vi "Configure A to B Sequence Trigger.vi"(0 "VISA resource name":refnum<visa-resource-name>, 1 "Enable B Trigger (T: Enable)":bool=TRUE, 2 "Trigger Reset Type (0:None)":u16(ring) items=["None", "Timeout", "State (Low)", "State (High)", "Transition (Rising)", "Transition (Falling)"], 5 "Trigger Mode (0:Trig After Time)":u16(ring) items=["Trig After Time", "Trig On nth Event"], 7 "Trigger Delay Time (6.0ns)":dbl=6e-09, 9 "Trigger Event (1)":i32=1, 11 "error in (no error)":errorcluster, 12 "Timeout (1.0Ms)":dbl=1000000.0, 13 "Source (0:Channel1)":u16(ring) items=["Channel1"=0, "Channel2"=1, "Channel3"=2, "Channel4"=3, "Aux"=12], 14 "Threshold (0.0v)":dbl) -> (4 "VISA resource name out":refnum<visa-resource-name>, 15 "error out":errorcluster)   [LabVIEW 2015, in "Tektronix 7000 Series.lvlib"]
doc: "Configures A to B Sequence. B trigger occurs after the main trigger event. It is available only when you enable B Trigger Type.\n\n<B>Note:</B> Not all models support all parameters contained in this VI. These settings are ignored by the driver if not supported.\n\nThis VI has been obsoleted from the driver and is included for compatibility with existing applications. New applications should use the Configure Trigger (A to B Sequence Mode) VI"
uses:
  <instrlib>/Tektronix 7000 Series/Tektronix 7000 Series.lvlib
panel:
  # "Note:\nThis VI has been obsoleted from the driver and is included for compatibility with existing applications.  New applications should use the Configure Trigger (A to B Sequence Mode) VI"
  # "Trigger Reset"
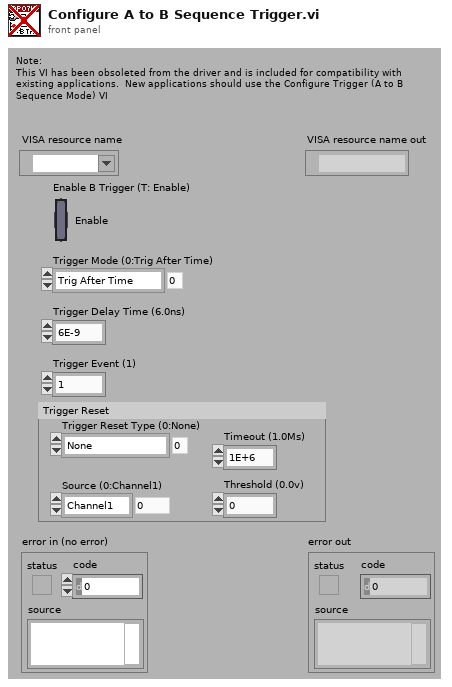
[diagram p1: front panel]
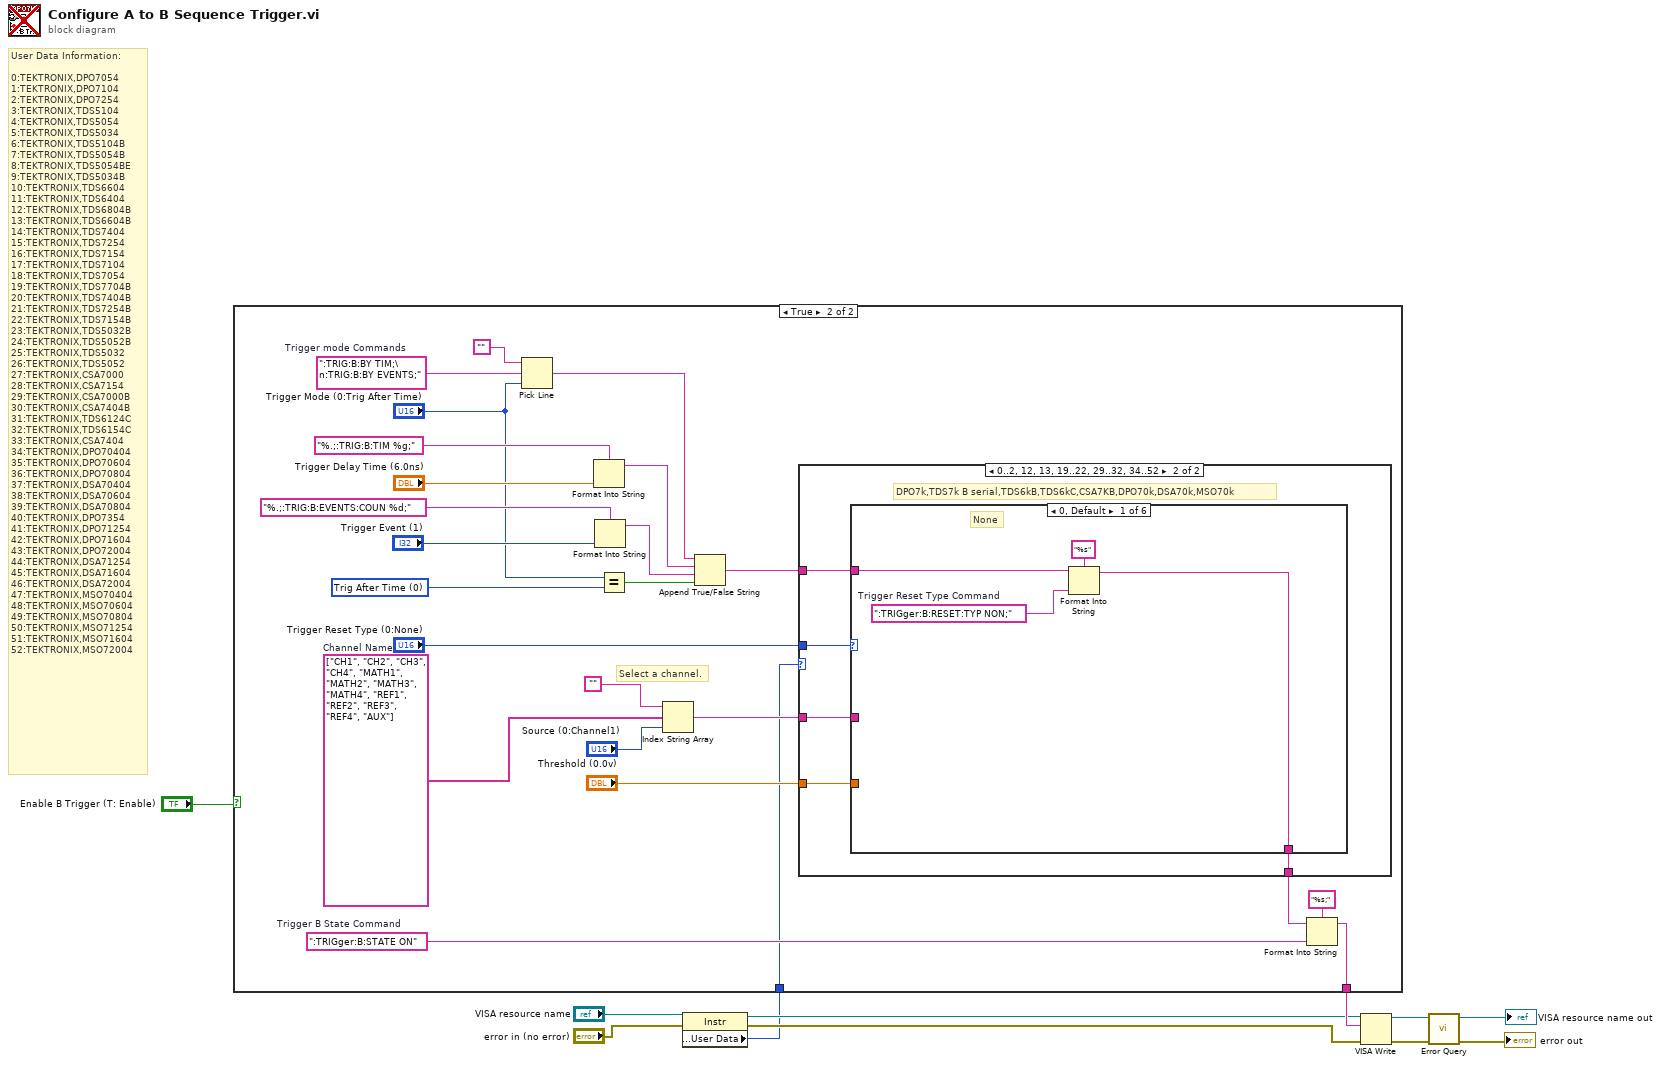
[diagram p0: block diagram]
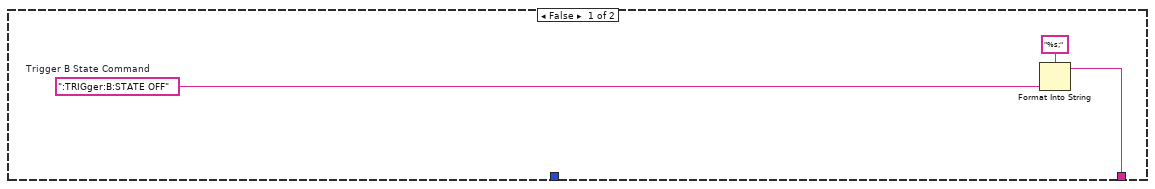
[diagram p2: hidden frame]
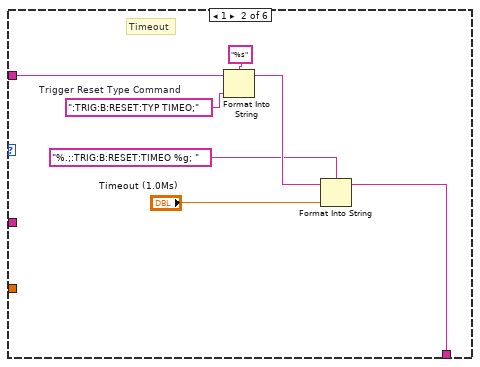
[diagram p4: hidden frame]
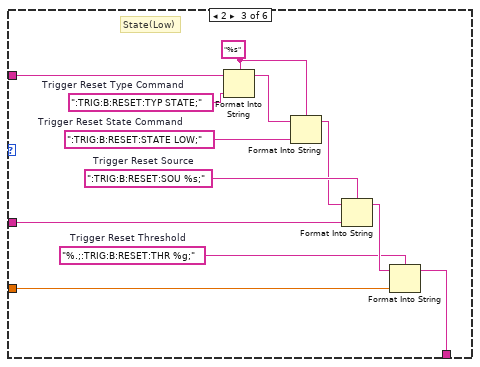
[diagram p5: hidden frame]
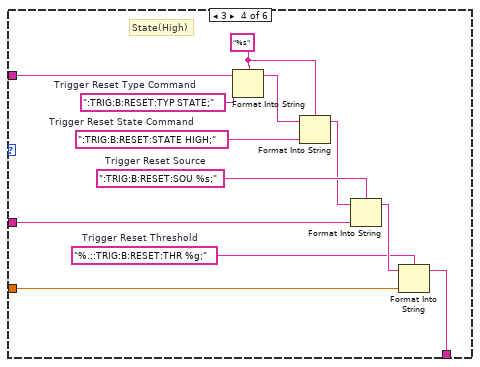
[diagram p6: hidden frame]
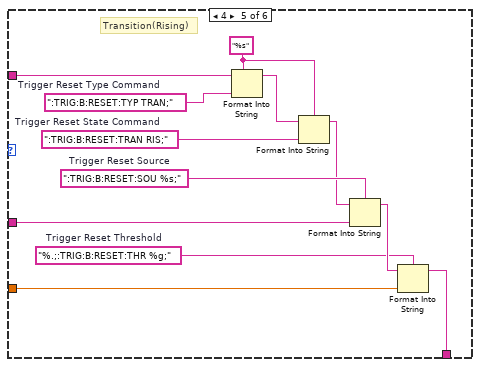
[diagram p7: hidden frame]
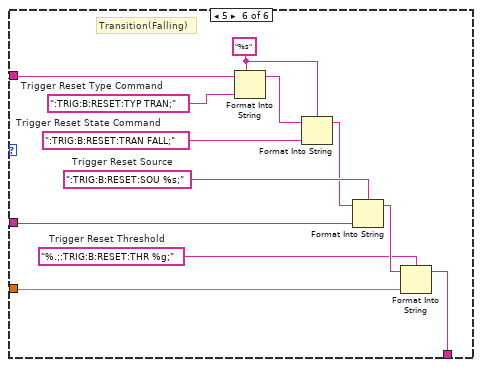
[diagram p8: hidden frame]
diagram:
  # "User Data Information:\n\n0:TEKTRONIX,DPO7054\n1:TEKTRONIX,DPO7104\n2:TEKTRONIX,DPO7254\n3:TEKTRONIX,TDS5104\n4:TEKTRONIX,TDS5054\n5:TEKTRONIX,TDS5034\n6:TEKTRONIX,TDS5104B\n7:TEKTRONIX,TDS5054B\n8:TEKTRONIX,TDS5054BE\n9:TEKTRONIX,TDS5034B\n10:TEKTRONIX,TDS6604\n11:TEKTRONIX,TDS6404\n12:TEKTRONIX,TDS6804B\n13:TEKTRONIX,TDS6604B\n14:TEKTRONIX,TDS7404\n15:TEKTRONIX,TDS7254\n16:TEKTRONIX,TDS7154\n17:TEKTRONIX,TDS7104\n18:TEKTRONIX,TDS7054\n19:TEKTRONIX,TDS7704B\n20:TEKTRONIX,TDS7404B\n21:TEKTRONIX,TDS7254B\n22:TEKTRONIX,TDS7154B\n23:TEKTRONIX,TDS5032B\n24:TEKTRONIX,TDS5052B\n25:TEKTRONIX,TDS5032\n26:TEKTRONIX,TDS5052\n27:TEKTRONIX,CSA7000\n28:TEKTRONIX,CSA7154\n29:TEKTRONIX,CSA7000B\n30:TEKTRONIX,CSA7404B\n31:TEKTRONIX,TDS6124C\n32:TEKTRONIX,TDS6154C\n33:TEKTRONIX,CSA7404\n34:TEKTRONIX,DPO70404\n35:TEKTRONIX,DPO70604\n36:TEKTRONIX,DPO70804\n37:TEKTRONIX,DSA70404\n38:TEKTRONIX,DSA70604\n39:TEKTRONIX,DSA70804\n40:TEKTRONIX,DPO7354\n41:TEKTRONIX,DPO71254\n42:TEKTRONIX,DPO71604\n43:TEKTRONIX,DPO72004\n44:TEKTRONIX,DSA71254\n45:TEKTRONIX,DSA71604\n46:TEKTRONIX,DSA72004\n47:TEKTRONIX,MSO70404\n48:TEKTRONIX,MSO70604\n49:TEKTRONIX,MSO70804\n50:TEKTRONIX,MSO71254\n51:TEKTRONIX,MSO71604\n52:TEKTRONIX,MSO72004"
  n1 = property class="Instr"(reference="VISA resource name", error in="error in (no error)") -> (reference out=w3:refnum<visa-resource-name>, error out=w2:errorcluster, "General Settings:User Data"=w1:u32)
  n2 = case shown="True" "Enable B Trigger (T: Enable)" {
    tunnel: [w12 w16] -> w7
    tunnel: w1 -> [_ w15]
    frame False {
      w14 = ":TRIGger:B:STATE OFF"  # Trigger B State Command
      n3 = Format Into String(format string="%s;", w14) -> (resulting string=w12:string)  [unwired: 2 in, 1 out]
    }
    frame True {
      w18 = ":TRIGger:B:STATE ON"  # Trigger B State Command
      w24 = string[] ["CH1", "CH2", "CH3", "CH4", "MATH1", "MATH2", "MATH3", "MATH4", "REF1", "REF2", "REF3", "REF4", "AUX"]  # Channel Name
      w32 = u16 0 items=["Trig After Time", "Trig On nth Event"] ("Trigger mode (0:Trig After Time)")
      w38 = ":TRIG:B:BY TIM;\n:TRIG:B:BY EVENTS;"  # Trigger mode Commands
      # "Select a channel."
      n4 = Pick Line(string ("")="" ("Empty String Constant"), multi-line string=w38, line index="Trigger Mode (0:Trig After Time)") -> (output string=w27:string)
      n5 = Format Into String(format string="%.;:TRIG:B:TIM %g;", "Trigger Delay Time (6.0ns)") -> (resulting string=w29:string)  [unwired: 2 in, 1 out]
      n6 = Format Into String(format string="%.;:TRIG:B:EVENTS:COUN %d;", "Trigger Event (1)") -> (resulting string=w28:string)  [unwired: 2 in, 1 out]
      n7 = Equal?(x="Trigger Mode (0:Trig After Time)", y=w32) -> (x = y?=w30:bool)
      n8 = Index String Array(1:"Source (0:Channel1)", 2:w24, 3:"" ("Empty String Constant")) -> (0:w21:string)
      n9 = Append True/False String(1:w30, 2:w28, 3:w29, 4:w27) -> (0:w25:string)
      n10 = case shown="0..2, 12, 13, 19..22, 29..32, 34..52" w15 {
        tunnel: "Trigger Reset Type (0:None)" -> [_ w44]
        tunnel: w25 -> [w39 w43]
        tunnel: w21 -> [_ w42]
        tunnel: "Threshold (0.0v)" -> [_ w41]
        tunnel: [w39 w40] -> w17
        frame Default {
        }
        frame 0..2, 12, 13, 19..22, 29..32, 34..52 {
          # "DPO7k,TDS7k B serial,TDS6kB,TDS6kC,CSA7KB,DPO70k,DSA70k,MSO70k"
          n11 = case shown="0, Default" w44 {
            tunnel: w43 -> [w47 w52 w66 w73 w83 w94]
            tunnel: w42 -> [_ _ w61 w72 w81 w93]
            tunnel: w41 -> [_ _ w58 w71 w82 w95]
            tunnel: [w45 w49 w56 w69 w80 w92] -> w40
            frame 0, Default {
              w46 = ":TRIGger:B:RESET:TYP NON;"  # Trigger Reset Type Command
              # "None"
              n12 = Format Into String(format string="%s", initial string=w47, w46) -> (resulting string=w45:string)  [unwired: 1 in, 1 out]
            }
            frame 1 {
              w53 = ":TRIG:B:RESET:TYP TIMEO;"  # Trigger Reset Type Command
              # "Timeout"
              n13 = Format Into String(format string="%s", initial string=w52, w53) -> (resulting string=w51:string)  [unwired: 1 in, 1 out]
              n14 = Format Into String(format string="%.;:TRIG:B:RESET:TIMEO %g; ", initial string=w51, "Timeout (1.0Ms)") -> (resulting string=w49:string)  [unwired: 1 in, 1 out]
            }
            frame 2 {
              w57 = "%.;:TRIG:B:RESET:THR %g;"  # Trigger Reset Threshold
              w64 = ":TRIG:B:RESET:STATE LOW;"  # Trigger Reset State Command
              w62 = ":TRIG:B:RESET:SOU %s;"  # Trigger Reset Source
              w65 = "%s" ("format string")
              w67 = ":TRIG:B:RESET:TYP STATE;"  # Trigger Reset Type Command
              # "State(Low)"
              n15 = Format Into String(format string=w65, initial string=w66, w67) -> (resulting string=w63:string)  [unwired: 1 in, 1 out]
              n16 = Format Into String(format string=w65, initial string=w63, w64) -> (resulting string=w60:string)  [unwired: 1 in, 1 out]
              n17 = Format Into String(format string=w62, initial string=w60, w61) -> (resulting string=w59:string)  [unwired: 1 in, 1 out]
              n18 = Format Into String(format string=w57, initial string=w59, w58) -> (resulting string=w56:string)  [unwired: 1 in, 1 out]
            }
            frame 3 {
              w74 = "%.;:TRIG:B:RESET:THR %g;"  # Trigger Reset Threshold
              w79 = ":TRIG:B:RESET:STATE HIGH;"  # Trigger Reset State Command
              w77 = ":TRIG:B:RESET:SOU %s;"  # Trigger Reset Source
              w70 = "%s" ("format string")
              w68 = ":TRIG:B:RESET:TYP STATE;"  # Trigger Reset Type Command
              # "State(High)"
              n19 = Format Into String(format string=w70, initial string=w73, w68) -> (resulting string=w78:string)  [unwired: 1 in, 1 out]
              n20 = Format Into String(format string=w70, initial string=w78, w79) -> (resulting string=w76:string)  [unwired: 1 in, 1 out]
              n21 = Format Into String(format string=w77, initial string=w76, w72) -> (resulting string=w75:string)  [unwired: 1 in, 1 out]
              n22 = Format Into String(format string=w74, initial string=w75, w71) -> (resulting string=w69:string)  [unwired: 1 in, 1 out]
            }
            frame 4 {
              w84 = "%.;:TRIG:B:RESET:THR %g;"  # Trigger Reset Threshold
              w89 = ":TRIG:B:RESET:TRAN RIS;"  # Trigger Reset State Command
              w87 = ":TRIG:B:RESET:SOU %s;"  # Trigger Reset Source
              w91 = "%s" ("format string")
              w90 = ":TRIG:B:RESET:TYP TRAN;"  # Trigger Reset Type Command
              # "Transition(Rising)"
              n23 = Format Into String(format string=w91, initial string=w83, w90) -> (resulting string=w88:string)  [unwired: 1 in, 1 out]
              n24 = Format Into String(format string=w91, initial string=w88, w89) -> (resulting string=w86:string)  [unwired: 1 in, 1 out]
              n25 = Format Into String(format string=w87, initial string=w86, w81) -> (resulting string=w85:string)  [unwired: 1 in, 1 out]
              n26 = Format Into String(format string=w84, initial string=w85, w82) -> (resulting string=w80:string)  [unwired: 1 in, 1 out]
            }
            frame 5 {
              w96 = "%.;:TRIG:B:RESET:THR %g;"  # Trigger Reset Threshold
              w101 = ":TRIG:B:RESET:TRAN FALL;"  # Trigger Reset State Command
              w99 = ":TRIG:B:RESET:SOU %s;"  # Trigger Reset Source
              w103 = "%s" ("format string")
              w102 = ":TRIG:B:RESET:TYP TRAN;"  # Trigger Reset Type Command
              # "Transition(Falling)"
              n27 = Format Into String(format string=w103, initial string=w94, w102) -> (resulting string=w100:string)  [unwired: 1 in, 1 out]
              n28 = Format Into String(format string=w103, initial string=w100, w101) -> (resulting string=w98:string)  [unwired: 1 in, 1 out]
              n29 = Format Into String(format string=w99, initial string=w98, w93) -> (resulting string=w97:string)  [unwired: 1 in, 1 out]
              n30 = Format Into String(format string=w96, initial string=w97, w95) -> (resulting string=w92:string)  [unwired: 1 in, 1 out]
            }
          }
        }
      }
      n31 = Format Into String(format string="%s;", initial string=w17, w18) -> (resulting string=w16:string)  [unwired: 1 in, 1 out]
    }
  }
  n32 = VISA Write(VISA resource name=w3, write buffer=w7, error in (no error)=w2) -> (VISA resource name out=w11:refnum<visa-resource-name>, error out=w10:errorcluster)  [unwired: 1 out]
  n33 = call <instrlib>:"Error Query.vi"("error in (no error)"=w10, "VISA resource name"=w11) -> ("error out"=→"error out":errorcluster, "VISA resource name out"=→"VISA resource name out":refnum<visa-resource-name>)  [unwired: 6 in, 2 out]
